vi "close.vi"(8 "error in":errorcluster, 11 "SQLite runtime in":refnum<class "SQLite runtime.lvclass">) -> (0 "error out":errorcluster)   [LabVIEW 2014, in "SQLite runtime.lvclass"]
doc: "Provides an interface for terminating a module instance. While this interface performs no operations, a child should close and deallocate any open references or memory."
uses:
  SQLite runtime.lvclass
  SQLite runtime.lvclass/SQLite runtime.ctl
  <vilib>/drjdpowell/SQLite Library/SQL Statement/SQL Statement.lvclass/SQL Statement.ctl
  <vilib>/drjdpowell/SQLite Library/SQL Connection/Connection.lvclass
  <vilib>/drjdpowell/SQLite Library/SQL Statement/SQL Statement.lvclass
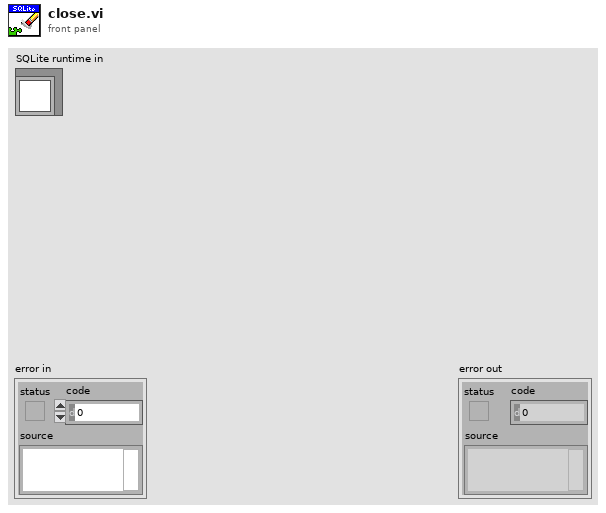
[diagram p1: front panel]
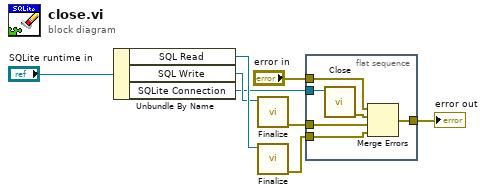
[diagram p0: block diagram]
diagram:
  n1 = Unbundle By Name("SQLite runtime in") -> ("SQL Read"=w7:refnum<class "SQL Statement.lvclass">, "SQL Write"=w6:refnum<class "SQL Statement.lvclass">, "SQLite Connection"=w5:refnum<class "Connection.lvclass">)
  n2 = call <vilib>:"Finalize.vi"("SQL Statement in"=w6) -> ("error out"=w3:errorcluster)  [unwired: 10 in]
  n3 = call <vilib>:"Finalize.vi"("SQL Statement in"=w7) -> ("error out"=w2:errorcluster)  [unwired: 10 in]
  n4 = flat-sequence {
    tunnel: w5 -> [w14]
    tunnel: [w13] -> w4
    tunnel: w3 -> [w11]
    tunnel: w2 -> [w10]
    tunnel: "error in" -> [w9]
    frame #0 {
      n5 = call-dynamic "Close.vi"("SQLite Connection in"=w14) -> ("error out"=w12:errorcluster)  [unwired: 10 in]
      n6 = Merge Errors(w9, w12, w11, w10) -> (w13:errorcluster)
    }
  }
  "error out" <- w4
